vi "Hill Equation.vi"(9 "K_a":dbl, 10 "n":dbl, 11 "input":dbl) -> (3 "output":dbl)   [LabVIEW 2014]
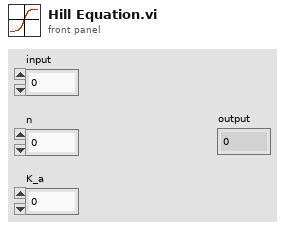
[diagram p1: front panel]
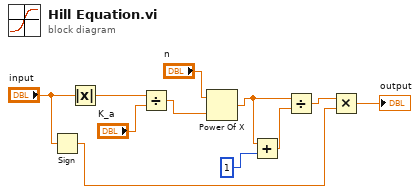
[diagram p0: block diagram]
diagram:
  n1 = Sign(1:"input") -> (0:w2:dbl)
  n2 = Absolute Value(x="input") -> (abs(x)=w10:dbl)
  n3 = Divide(x=w10, y="K_a") -> (x/y=w4:dbl)
  n4 = Power Of X(1:w4, 2:"n") -> (0:w8:dbl)
  n5 = Add(x=w8, y=1) -> (x+y=w6:dbl)
  n6 = Divide(x=w8, y=w6) -> (x/y=w3:dbl)
  n7 = Multiply(x=w3, y=w2) -> (x*y=→"output":dbl)
